vi "MacroExecution and Timing.vi"(7 "MacroExecution and Timing Command":T3, 8 "Error In":errorcluster, 10 "Index IN":i32, 11 "Macro IN":string[](array[string])) -> (0 "Error Out":errorcluster, 1 "Estimated Timing cluster":T1, 2 "Pause Duration":dbl, 3 "Execution Status":T2=enum."Skip", 4 "Current Command":string, 5 "Current Execution Index":i32)   [LabVIEW 2012]
doc: "SciScan 1.2 160622"
uses:
  Macro Execution and Timing_Commands.ctl
  Custom Controls and Typedefs/ExecutionStatus.ctl
  Estimated Timing Cluster.ctl
  Custom Controls/MAIN Image panel tab Control type def.ctl
  MacroGUI Module/Custom Controls and Typedefs/LOOP Control Cluster.ctl
  Custom Controls/Stage Position Data.ctl
  Custom Controls/file format type def.ctl
  GFG/GFGbooleanGet.vi
  GFG/GFGpathGet.vi
  GFG/GFG library.lvlib
panel:
  out "Step time array":dbl[](array[numeric])
  out "Remaining/Estimated Run Time":dbl
  out "Skip?":bool
  out "Paused?":bool
  out "Execution Complete?":bool
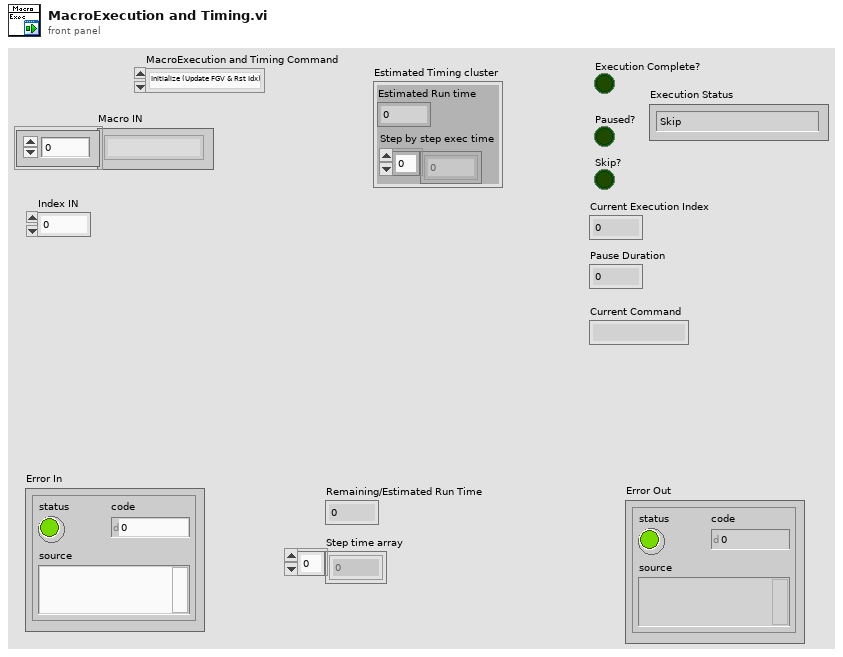
[diagram p1: front panel]
types:
  T1 = typedef "Estimated Timing Cluster.ctl" = cluster{"Estimated Run time":dbl, "Step by step exec time":dbl[]}
  T2 = typedef "ExecutionStatus.ctl" = enum16{"Instruction Available", "Skip", "Exec Paused", "Exec Complete", "Exec Waiting for Trigger"}
  T3 = typedef "Macro Execution and Timing_Commands.ctl" = enum16{"Initialize (Update FGV & Rst Idx)", "Run", "EstimateTime", "Preview", "Update Macro array (Idx Unchanged)", "Update Index", "Clear Timing Info"}
  T4 = typedef "MAIN Image panel tab Control type def.ctl" = enum32{"Channel 1", "Channel 2", "Channel 3", "Channel 4", "all channels", "RGB overlay", "ROI", "arbitrary line scan"}
  T5 = typedef "LOOP Control Cluster.ctl" = cluster{"Index of LOOP.Start":i32, "Iteration Count Down":i32, "No of iterations (N)":i32}
  T6 = typedef "file format type def.ctl" = enum16{"16bit raw", "32bit raw", "16bit multi-tiff (interleave)", "16bit multi-tiff (separate)", "16bit multi-tiff (stacked)", "32bit multi-tiff (interleave)", "32bit multi-tiff (separate)", "32bit multi-tiff (stacked)", "16bit tiff series (interleave)", "16bit tiff series (separate)", "16bit tiff series (stacked)", "32bit tiff series (interleave)", "32bit tiff series (separate)", "32bit tiff series (stacked)"}
  T7 = typedef "Stage Position Data.ctl" = cluster{"X":dbl, "Y":dbl, "Z":dbl}
  T8 = typedef "Macro_Action_List.ctl" = enum16{"Unknown Command", "2D.Frame.Scan", "2D.Line.Scan", "Load.Settings.File", "Move.To.Position", "Pause", "Z.Stack", "LOOP.Start", "LOOP.End", "Record", "Fast.Z", "Generic", "Slow.Z", "Tiling", "Preset.End"}
  T9 = typedef "VariantType.lvlib/Type.ctl" = enum8{"Invalid Type", "Void", "I8", "I16", "I32", "I64", "U8", "U16", "U32", "U64", "Single Float", "Double Float", "Extended Float", "Single Complex", "Double Complex", "Extended Complex", "Enum U8", "Enum U16", "Enum U32", "Enum U64", "Single Float With Unit", "Double Float With Unit", "Extended Float With Unit", "Single Complex with Unit", "Double Complex with Unit", "Extended Complex with Unit", "Boolean", "String", "Path", "Picture", "Tag", "Array", "Cluster", "Variant", "LV Variant", "Waveform", "Timestamp", "Digital Waveform", "Digital Data", "ExpressData", "Refnum", "External Data", "VI", "Poly VI", "LabVIEW Class Instance", "Fixed Point"}
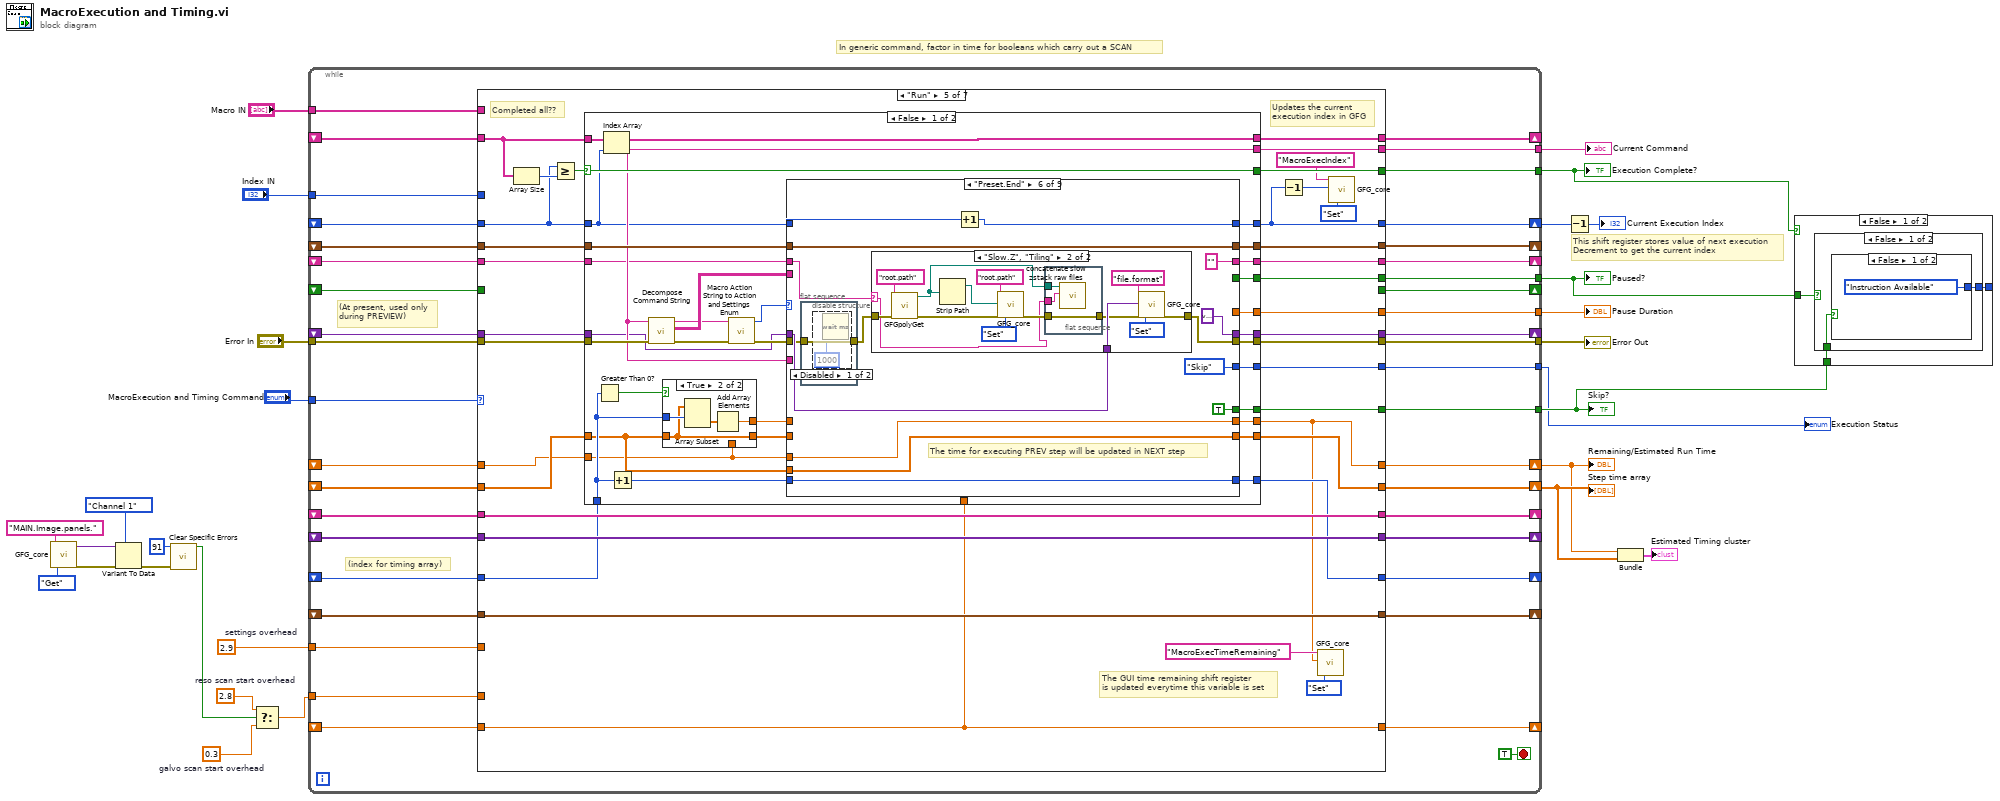
[diagram p0: block diagram]
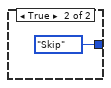
[diagram p2: hidden frame]
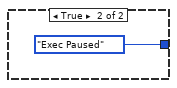
[diagram p3: hidden frame]
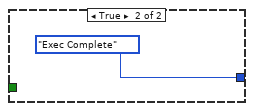
[diagram p4: hidden frame]
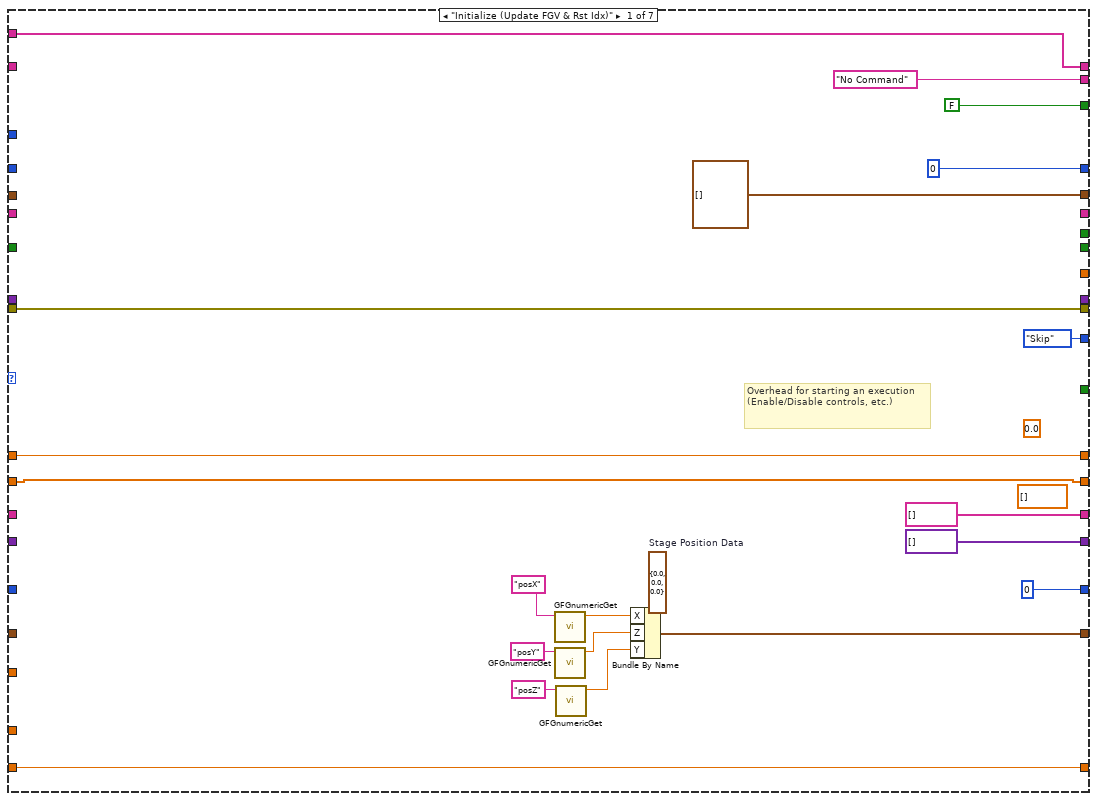
[diagram p5: hidden frame]
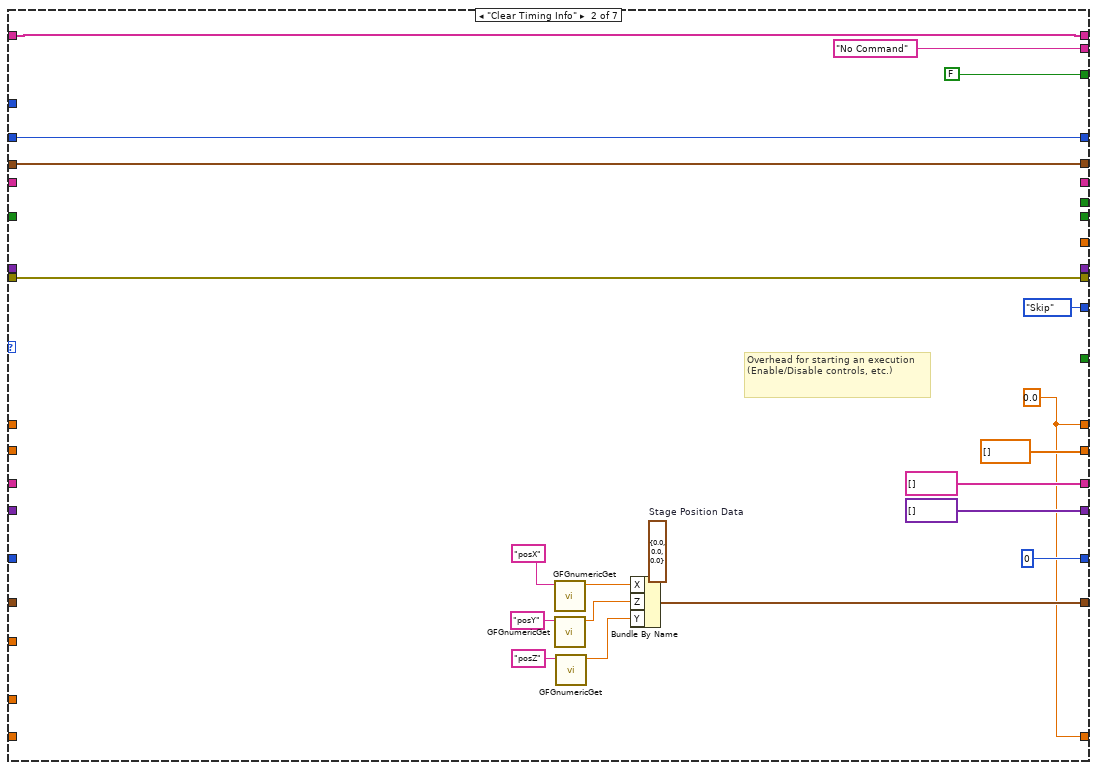
[diagram p6: hidden frame]
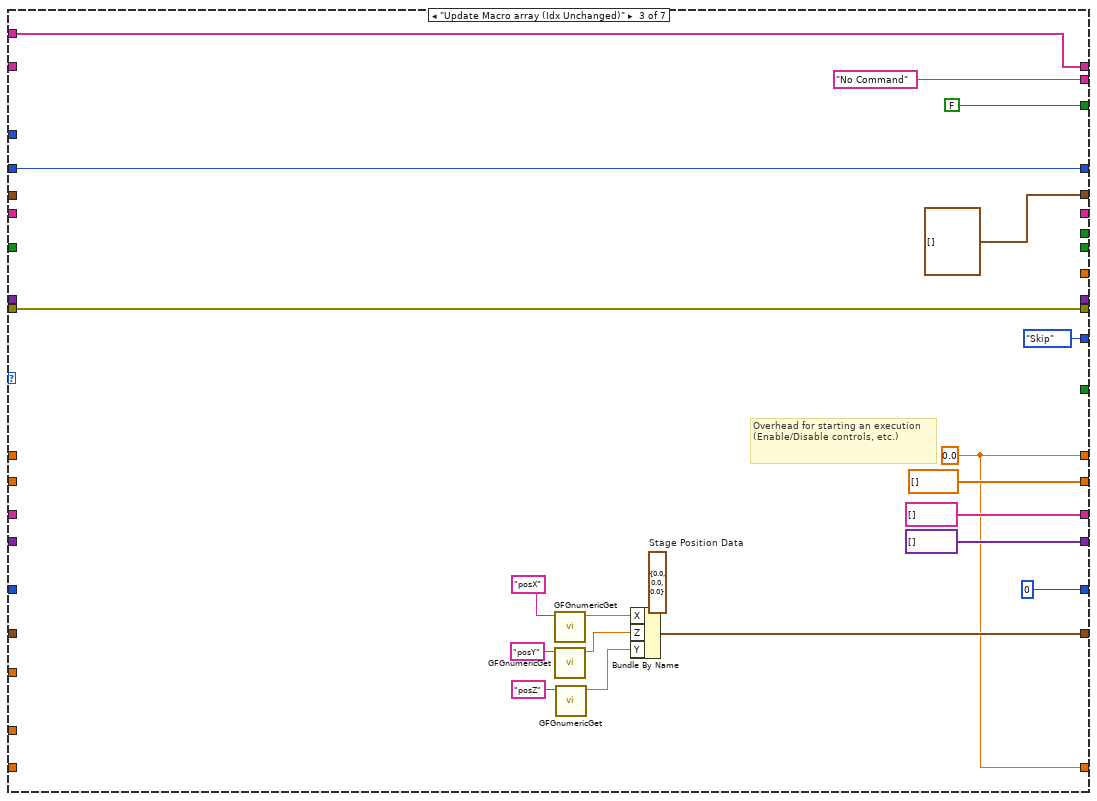
[diagram p7: hidden frame]
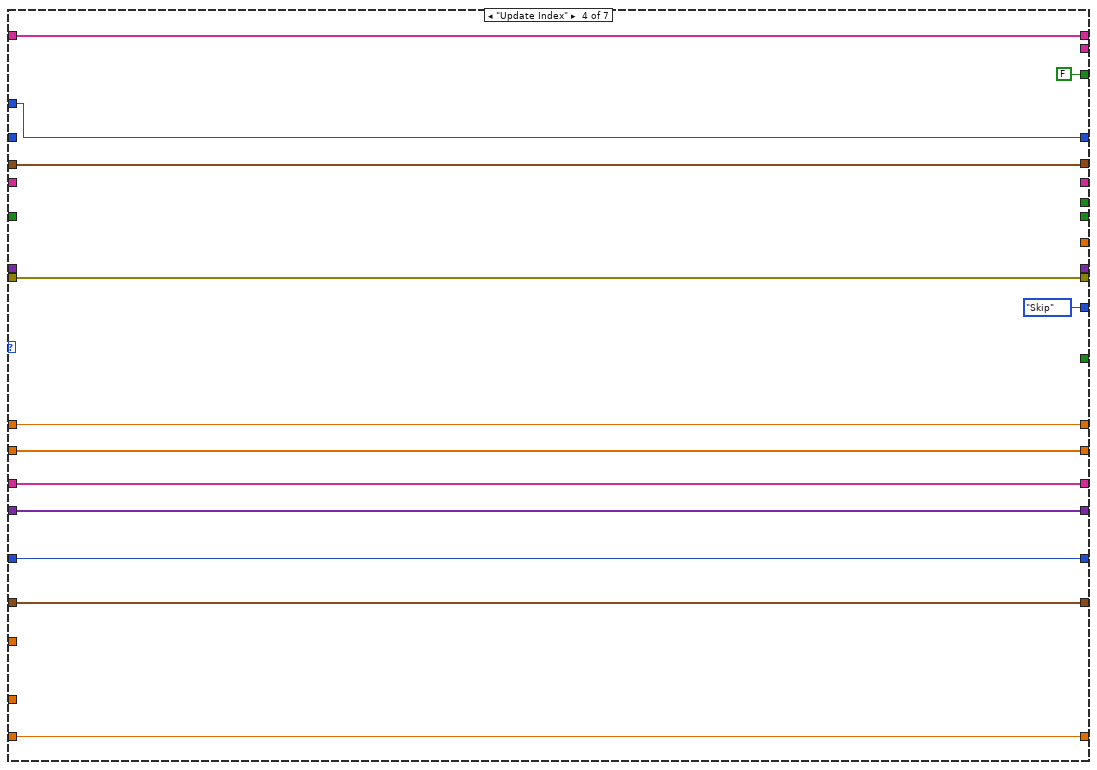
[diagram p8: hidden frame]
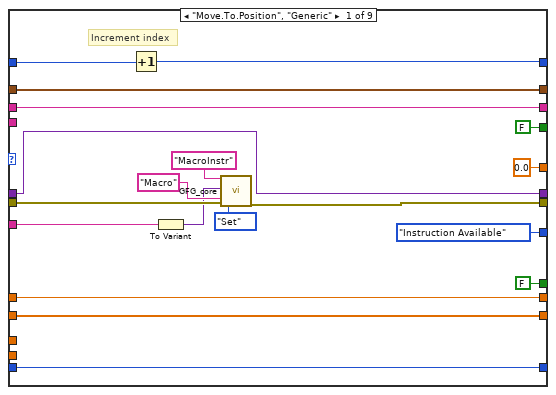
[diagram p10: hidden frame]
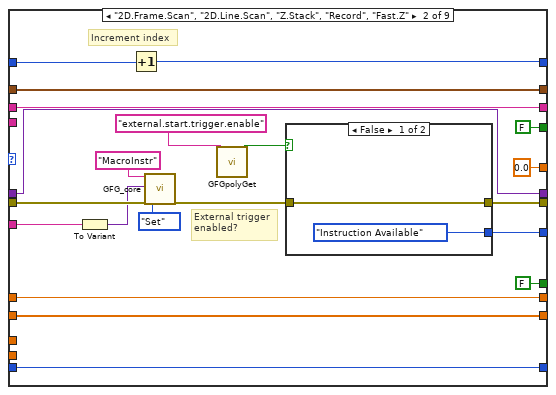
[diagram p11: hidden frame]
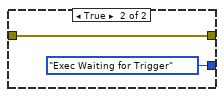
[diagram p12: hidden frame]
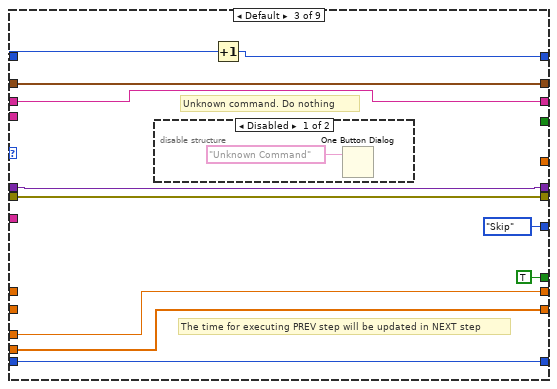
[diagram p13: hidden frame]
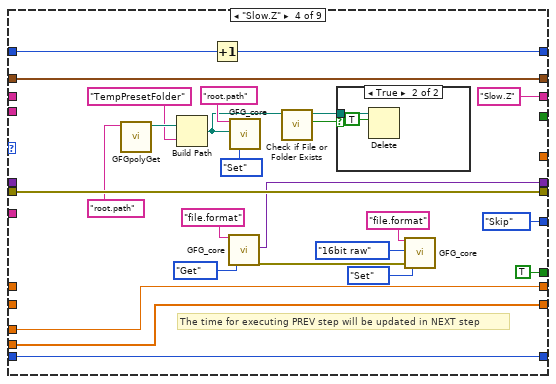
[diagram p15: hidden frame]
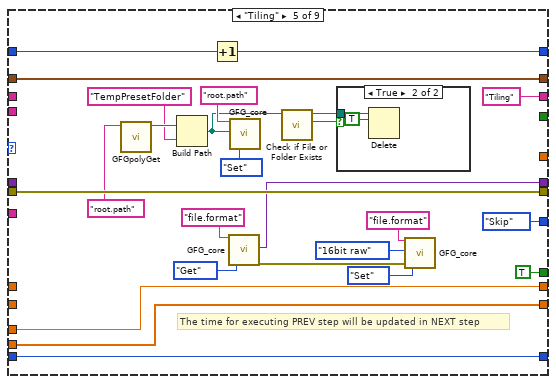
[diagram p17: hidden frame]
diagram:
  w9 = 0.3  # galvo scan start overhead
  w11 = 2.8  # reso scan start overhead
  w12 = 2.9  # settings overhead
  # "In generic command, factor in time for booleans which carry out a SCAN"
  # "This shift register stores value of next execution\nDecrement to get the current index"
  n1 = call "GFG_core.vi"("Variable Name in"="MAIN.Image.panels.", "Action"=enum16{"Init", "Set", "Get", "Clear"}."Get") -> ("Variant Out"=w5:variant, "error out"=w7:errorcluster)  [unwired: 11 in, 5 out]
  n2 = Variant To Data(error in=w7, type=MAIN_Image_panel_tab_Control_type_def."Channel 1" ("MAIN Image panels"), Variant=w5) -> (error out=w4:errorcluster)  [unwired: 1 out]
  n3 = call "Clear Specific Errors.vi"("Error In"=w4, "Error number In"=91) -> ("Error Cleared?"=w2:bool)  [unwired: 8 in, 1 out]
  n4 = Select(t=w11, s=w2, f=w9) -> (s? t:f=w10:dbl)
  n5 = while {
    shift-right: [w63] -> w24
    shift-left: _ -> [w68]
    tunnel: [w65] -> w22
    tunnel: "MacroExecution and Timing Command" -> [w64]
    shift-right: [w62] -> _
    shift-left: _ -> [w67]
    shift-right: [w60] -> _
    shift-left: _ -> [w61]
    tunnel: "Error In" -> [w59]
    tunnel: [w58] -> w26
    tunnel: [w57] -> w21
    tunnel: [w56] -> w25
    tunnel: [w55] -> w20
    tunnel: [w54] -> w23
    shift-right: [w53] -> w17
    shift-left: _ -> [w52]
    shift-right: [w51] -> w18
    shift-left: _ -> [w50]
    shift-right: [w49] -> _
    shift-left: _ -> [w47]
    shift-right: [w48] -> _
    shift-left: _ -> [w46]
    shift-right: [w45] -> _
    shift-left: _ -> [w44]
    shift-right: [w43] -> _
    shift-left: _ -> [w42]
    shift-right: [w41] -> _
    shift-left: _ -> [w40]
    tunnel: [w39] -> w15
    tunnel: "Macro IN" -> [w38]
    tunnel: "Index IN" -> [w37]
    tunnel: w12 -> [w36]
    tunnel: w10 -> [w35]
    shift-right: [w34] -> _
    shift-left: _ -> [w33]
    shift-right: [w32] -> _
    shift-left: _ -> [w31]
    shift-right: [w30] -> _
    shift-left: _ -> [w29]
    stop <- TRUE stop-if-true
    # "(At present, used only\nduring PREVIEW)"
    # "(index for timing array)"
    n6 = case shown="\"Run\"" w64 {
      tunnel: w68 -> [_ w92 w110 _ w176 w472 w907]
      tunnel: w67 -> [_ w94 _ w142 w175 w471 w920]
      tunnel: [FALSE FALSE FALSE FALSE w173 w469 w917] -> w65
      tunnel: [0 w92 w110 w139 w160 w464 w918] -> w63
      tunnel: [w72 w94 w111 w142 w172 w468 w920] -> w62
      tunnel: w61 -> [_ w93 _ w138 w171 w467 w911]
      tunnel: [T5[] [] w93 T5[] [] w138 w169 w465 w911] -> w60
      tunnel: w59 -> [w86 w108 w127 w137 w170 w466 w908]
      tunnel: [w86 w108 w127 w137 w168 w463 w910] -> w58
      tunnel: [_ _ _ _ w167 w462 _] -> w57
      tunnel: [_ _ _ _ w166 w461 _] -> w56
      tunnel: [_ _ _ _ w165 w460 _] -> w55
      tunnel: ["No Command" ("String") "No Command" ("String") "No Command" ("String") _ w164 w459 w916] -> w54
      tunnel: [w70 w90 w113 w141 w149 w458 w924] -> w53
      tunnel: w52 -> [w70 _ _ w141 w147 w457 w924]
      tunnel: [w71 dbl[] [] dbl[] [] w135 w154 w456 w923] -> w51
      tunnel: w50 -> [w71 _ _ w135 w156 w455 w923]
      tunnel: [string[] [] string[] [] string[] [] w134 w163 w452 w915] -> w49
      tunnel: [variant[] [] variant[] [] variant[] [] w133 w162 w451 w914] -> w48
      tunnel: w47 -> [_ _ _ w134 w163 w454 w915]
      tunnel: w46 -> [_ _ _ w133 w162 w453 w914]
      tunnel: [w75 w97 w115 w131 w161 w449 w912] -> w45
      tunnel: w44 -> [_ _ _ w131 w161 w450 w912]
      tunnel: [0 0 0 w132 w153 0 w913] -> w43
      tunnel: w42 -> [_ _ _ w132 w155 _ w913]
      tunnel: [w69 w90 w113 w130 w152 w448 w909] -> w41
      tunnel: w40 -> [w69 _ _ w130 w152 w447 w909]
      tunnel: [ExecutionStatus."Skip" ("Execution Status") ExecutionStatus."Skip" ("Execution Status") ExecutionStatus."Skip" ("Execution Status") ExecutionStatus."Skip" ("Execution Status") w148 w445 w919] -> w39
      tunnel: w38 -> [w72 _ w111 _ _ _ _]
      tunnel: w37 -> [_ _ _ w139 _ _ _]
      tunnel: w36 -> [_ _ _ _ _ w444 _]
      tunnel: w35 -> [_ _ _ _ _ w443 _]
      tunnel: [_ _ _ _ w146 _ _] -> w34
      tunnel: w33 -> [_ _ _ _ w145 _ _]
      tunnel: [_ _ _ _ w144 _ _] -> w32
      tunnel: w31 -> [_ _ _ _ w143 _ _]
      tunnel: [_ _ _ _ _ _ w906] -> w30
      tunnel: w29 -> [_ _ _ _ _ _ w905]
      frame "Initialize (Update FGV & Rst Idx)" {
        w79 = T7 {"X"=0.0, "Y"=0.0, "Z"=0.0}  # Stage Position Data
        (unwired) dbl[] []
        (unwired) 0.0 ("number")
        # "Overhead for starting an execution\n(Enable/Disable controls, etc.)"
        n7 = call "GFGnumericGet.vi"("Variable Name in"="posX" ("String")) -> ("Numeric"=w78:dbl)  [unwired: 8 in, 2 out]
        n8 = call "GFGnumericGet.vi"("Variable Name in"="posY" ("String")) -> ("Numeric"=w77:dbl)  [unwired: 8 in, 2 out]
        n9 = call "GFGnumericGet.vi"("Variable Name in"="posZ" ("String")) -> ("Numeric"=w76:dbl)  [unwired: 8 in, 2 out]
        n10 = Bundle By Name(cluster=w79, "X"=w78, "Z"=w77, "Y"=w76) -> (w75:T7)
      }
      frame "Clear Timing Info" {
        w101 = T7 {"X"=0.0, "Y"=0.0, "Z"=0.0}  # Stage Position Data
        w90 = 0.0 ("number")
        # "Overhead for starting an execution\n(Enable/Disable controls, etc.)"
        n11 = call "GFGnumericGet.vi"("Variable Name in"="posX" ("String")) -> ("Numeric"=w100:dbl)  [unwired: 8 in, 2 out]
        n12 = call "GFGnumericGet.vi"("Variable Name in"="posY" ("String")) -> ("Numeric"=w99:dbl)  [unwired: 8 in, 2 out]
        n13 = call "GFGnumericGet.vi"("Variable Name in"="posZ" ("String")) -> ("Numeric"=w98:dbl)  [unwired: 8 in, 2 out]
        n14 = Bundle By Name(cluster=w101, "X"=w100, "Z"=w99, "Y"=w98) -> (w97:T7)
      }
      frame "Update Macro array (Idx Unchanged)" {
        w119 = T7 {"X"=0.0, "Y"=0.0, "Z"=0.0}  # Stage Position Data
        w113 = 0.0 ("number")
        # "Overhead for starting an execution\n(Enable/Disable controls, etc.)"
        n15 = call "GFGnumericGet.vi"("Variable Name in"="posX" ("String")) -> ("Numeric"=w118:dbl)  [unwired: 8 in, 2 out]
        n16 = call "GFGnumericGet.vi"("Variable Name in"="posY" ("String")) -> ("Numeric"=w117:dbl)  [unwired: 8 in, 2 out]
        n17 = call "GFGnumericGet.vi"("Variable Name in"="posZ" ("String")) -> ("Numeric"=w116:dbl)  [unwired: 8 in, 2 out]
        n18 = Bundle By Name(cluster=w119, "X"=w118, "Z"=w117, "Y"=w116) -> (w115:T7)
      }
      frame "Update Index" {
      }
      frame "Run" {
        # "Updates the current\nexecution index in GFG"
        # "The GUI time remaining shift register\nis updated everytime this variable is set"
        # "Completed all??"
        n19 = Array Size(array=w175) -> (size(s)=w177:i32)
        n20 = Greater Or Equal?(x=w176, y=w177) -> (x >= y?=w174:bool)
        n21 = case shown="False" w174 {
          selector: w174 -> [w209 w441]
          tunnel: w176 -> [w197 w438]
          tunnel: w175 -> [w208 w442]
          tunnel: [w209 w441] -> w173
          tunnel: [w208 w442] -> w172
          tunnel: w171 -> [w206 w439]
          tunnel: w170 -> [w207 w440]
          tunnel: [w205 w439] -> w169
          tunnel: [w204 w438] -> w160
          tunnel: [w203 w440] -> w168
          tunnel: [w201 _] -> w167
          tunnel: [w200 _] -> w166
          tunnel: [w199 _] -> w165
          tunnel: [w198 "No Command" ("String")] -> w164
          tunnel: w156 -> [w187 w435]
          tunnel: w155 -> [w190 _]
          tunnel: [w196 w435] -> w154
          tunnel: [w195 w434] -> w149
          tunnel: [w194 0] -> w153
          tunnel: w152 -> [_ w434]
          tunnel: [w193 ExecutionStatus."Exec Complete" ("Execution Status")] -> w148
          tunnel: w147 -> [w186 _]
          tunnel: [w181 _] -> w146
          tunnel: w145 -> [w180 _]
          tunnel: [w179 _] -> w144
          tunnel: w143 -> [w178 _]
          frame False {
            n22 = Greater Than 0?(x=w190) -> (x > 0?=w191:bool)
            n23 = Index Array(array=w208, index=w197) -> (element=w198:string)
            n24 = Increment(x=w190) -> (x+1=w192:i32)
            n25 = call "Decompose Command String.vi"("Error In"=w207, "Command IN"=w198) -> ("Error Out"=w185:errorcluster, "Parameter Table"=w202:string[][], "Action"=w183:string)  [unwired: 6 in, 1 out]
            n26 = case shown="True" w191 {
              tunnel: w187 -> [w211 w213]
              tunnel: w190 -> [_ w215]
              tunnel: [w211 w213] -> w189
              tunnel: [w210 w212] -> w188
              tunnel: w186 -> [w210 _]
              frame False {
              }
              frame True {
                n27 = Array Subset(array=w213, index=w215) -> (w214:dbl[])  [unwired: 1 in]
                n28 = Add Array Elements(numeric array=w214) -> (sum=w212:dbl)
              }
            }
            n29 = call "Macro Action String to Action and Settings Enum.vi"("error in (no error)"=w185, "Action String IN"=w183) -> ("error out"=w184:errorcluster, "Action Enum OUT"=w182:T8)  [unwired: 6 in, 2 out]
            n30 = case shown="\"Preset.End\"" w182 {
              tunnel: w184 -> [w225 w247 w267 w293 w320 w327 w368 w390 w415]
              tunnel: w197 -> [w234 w255 w270 w296 w323 w340 w376 w392 w412]
              tunnel: w206 -> [w232 w253 w268 w294 w321 w338 w377 w395 w417]
              tunnel: [w232 w253 w268 w294 w321 w338 w377 w394 w416] -> w205
              tunnel: [w233 w254 w269 w295 w322 w339 w375 w391 w411] -> w204
              tunnel: [w222 w240 w267 w293 w320 w328 w368 w390 w415] -> w203
              tunnel: w198 -> [w224 w246 _ _ _ _ _ _ _]
              tunnel: w202 -> [_ _ _ _ _ _ w373 w389 _]
              tunnel: [FALSE FALSE _ _ _ _ TRUE _ _] -> w201
              tunnel: [0.0 0.0 _ _ _ _ w369 _ _] -> w200
              tunnel: [FALSE ("Skip?") FALSE ("Skip?") TRUE ("Skip?") TRUE ("Skip?") TRUE ("Skip?") TRUE ("Skip?") FALSE ("Skip?") TRUE ("Skip?") TRUE ("Skip?")] -> w199
              tunnel: w188 -> [w219 w238 _ _ _ _ w364 w381 w403]
              tunnel: w189 -> [w220 w239 _ _ _ _ w365 w382 w404]
              tunnel: [w220 w239 w263 w289 w316 w334 w365 w382 w404] -> w196
              tunnel: [w219 w238 w262 w288 w315 w333 w364 w381 w403] -> w195
              tunnel: [w218 w237 w264 w290 w317 w335 w363 w380 w402] -> w194
              tunnel: [ExecutionStatus."Instruction Available" ("Execution Status") w241 ExecutionStatus."Skip" ("Execution Status") ExecutionStatus."Skip" ("Execution Status") ExecutionStatus."Skip" ("Execution Status") ExecutionStatus."Skip" ("Execution Status") ExecutionStatus."Exec Paused" ("Execution Status") ExecutionStatus."Skip" ("Execution Status") ExecutionStatus."Skip" ("Execution Status")] -> w193
              tunnel: w192 -> [w218 w237 w264 w290 w317 w335 w363 w380 w402]
              tunnel: w187 -> [_ _ w263 w289 w316 w334 _ _ _]
              tunnel: w186 -> [_ _ w262 w288 w315 w333 _ _ _]
              tunnel: [w217 w236 w261 "Slow.Z" ("Variable Name in") "Tiling" ("Variable Name in") "" ("Variable Name in") w362 w379 w401] -> w181
              tunnel: w180 -> [w217 w236 w261 _ _ w331 w362 w379 w401]
              tunnel: [w216 w235 w260 w276 w303 variant ("Variant Out") w361 w378 w400] -> w179
              tunnel: w178 -> [w216 w235 w260 _ _ w329 w361 w378 w400]
              frame "Move.To.Position", "Generic" {
                # "Increment index"
                n31 = Increment(x=w234) -> (x+1=w233:i32)
                n32 = To Variant(anything=w224) -> (Variant=w223:variant)
                n33 = call "GFG_core.vi"("Variable Name in"="MacroInstr" ("Source VI"), "Variant in"=w223, "Source VI"="Macro", "error in (no error)"=w225, "Action"=enum16{"Init", "Set", "Get", "Clear"}."Set") -> ("error out"=w222:errorcluster)  [unwired: 8 in, 6 out]
              }
              frame "2D.Frame.Scan", "2D.Line.Scan", "Z.Stack", "Record", "Fast.Z" {
                # "External trigger \nenabled?"
                # "Increment index"
                n34 = To Variant(anything=w246) -> (Variant=w245:variant)
                n35 = Increment(x=w255) -> (x+1=w254:i32)
                n36 = call "GFG_core.vi"("Variable Name in"="MacroInstr" ("Source VI"), "Variant in"=w245, "error in (no error)"=w247, "Action"=enum16{"Init", "Set", "Get", "Clear"}."Set") -> ("error out"=w242:errorcluster)  [unwired: 9 in, 6 out]
                n37 = call-poly "GFGpolyGet.vi"("Variable Name in"="external.start.trigger.enable") -> ("Boolean Value OUT"=w243:bool)  [unwired: 9 in, 1 out]
                n38 = case shown="False" w243 {
                  tunnel: w242 -> [w256 w258]
                  tunnel: [ExecutionStatus."Instruction Available" ("Execution Status") ExecutionStatus."Exec Waiting for Trigger" ("Execution Status")] -> w241
                  tunnel: [w256 w258] -> w240
                  frame False {
                  }
                  frame True {
                  }
                }
              }
              frame Default {
                # "The time for executing PREV step will be updated in NEXT step"
                # "Unknown command. Do nothing"
                n39 = disable-structure shown="Disabled" {
                  frame Disabled {
                    n40 = One Button Dialog(message="Unknown Command") -> ()  [unwired: 1 in, 1 out]
                  }
                  frame Enabled {
                  }
                }
                n41 = Increment(x=w270) -> (x+1=w269:i32)
              }
              frame "Slow.Z" {
                # "The time for executing PREV step will be updated in NEXT step"
                n42 = call-poly "GFGpolyGet.vi"("Variable Name in"="root.path") -> ("Path"=w283:path)  [unwired: 8 in, 2 out]
                n43 = Build Path(base path=w283, name or relative path="TempPresetFolder") -> (appended path=w274:path)
                n44 = Increment(x=w296) -> (x+1=w295:i32)
                n45 = call "GFG_core.vi"("Variable Name in"="file.format", "Action"=enum16{"Init", "Set", "Get", "Clear"}."Get") -> ("Variant Out"=w276:variant, "error out"=w275:errorcluster)  [unwired: 11 in, 5 out]
                n46 = call "GFG_core.vi"("Variable Name in"="root.path", "Variant in"=w274, "Action"=enum16{"Init", "Set", "Get", "Clear"}."Set") -> ()  [unwired: 10 in, 7 out]
                n47 = call <vilib>:"Check if File or Folder Exists.vi"("path"=w274) -> ("file or folder exists?"=w273:bool, "dup path"=w272:path)  [unwired: 8 in, 1 out]
                n48 = case shown="True" w273 {
                  tunnel: w272 -> [_ w298]
                  frame False {
                  }
                  frame True {
                    n49 = Delete(path (use dialog)=w298, entire hierarchy (F)=TRUE) -> ()  [unwired: 3 in, 3 out]
                  }
                }
                n50 = call "GFG_core.vi"("Variable Name in"="file.format", "Variant in"=file_format_type_def."16bit raw" ("file format"), "error in (no error)"=w275, "Action"=enum16{"Init", "Set", "Get", "Clear"}."Set") -> ()  [unwired: 9 in, 7 out]
              }
              frame "Tiling" {
                # "The time for executing PREV step will be updated in NEXT step"
                n51 = call-poly "GFGpolyGet.vi"("Variable Name in"="root.path") -> ("Path"=w310:path)  [unwired: 8 in, 2 out]
                n52 = Build Path(base path=w310, name or relative path="TempPresetFolder") -> (appended path=w301:path)
                n53 = Increment(x=w323) -> (x+1=w322:i32)
                n54 = call "GFG_core.vi"("Variable Name in"="file.format", "Action"=enum16{"Init", "Set", "Get", "Clear"}."Get") -> ("Variant Out"=w303:variant, "error out"=w302:errorcluster)  [unwired: 11 in, 5 out]
                n55 = call "GFG_core.vi"("Variable Name in"="root.path", "Variant in"=w301, "Action"=enum16{"Init", "Set", "Get", "Clear"}."Set") -> ()  [unwired: 10 in, 7 out]
                n56 = call <vilib>:"Check if File or Folder Exists.vi"("path"=w301) -> ("file or folder exists?"=w300:bool, "dup path"=w299:path)  [unwired: 8 in, 1 out]
                n57 = case shown="True" w300 {
                  tunnel: w299 -> [_ w325]
                  frame False {
                  }
                  frame True {
                    n58 = Delete(path (use dialog)=w325, entire hierarchy (F)=TRUE) -> ()  [unwired: 3 in, 3 out]
                  }
                }
                n59 = call "GFG_core.vi"("Variable Name in"="file.format", "Variant in"=file_format_type_def."16bit raw" ("file format"), "error in (no error)"=w302, "Action"=enum16{"Init", "Set", "Get", "Clear"}."Set") -> ()  [unwired: 9 in, 7 out]
              }
              frame "Preset.End" {
                # "The time for executing PREV step will be updated in NEXT step"
                n60 = flat-sequence {
                  tunnel: w327 -> [w341]
                  tunnel: [w341] -> w326
                  frame #0 {
                    n61 = disable-structure shown="Disabled" {
                      frame Disabled {
                        n62 = Wait (ms)(milliseconds to wait=u32 1000) -> ()  [unwired: 1 out]
                      }
                      frame Enabled {
                      }
                    }
                  }
                }
                n63 = case shown="\"Slow.Z\", \"Tiling\"" w331 {
                  selector: w331 -> [_ w344]
                  tunnel: w329 -> [_ w348]
                  tunnel: [w343 w346] -> w328
                  tunnel: w326 -> [w343 w345]
                  frame Default {
                  }
                  frame "Slow.Z", "Tiling" {
                    n64 = call-poly "GFGpolyGet.vi"("error in (no error)"=w345, "Variable Name in"="root.path") -> ("error out"=w357:errorcluster, "Path"=w351:path)  [unwired: 7 in, 1 out]
                    n65 = Strip Path(path=w351) -> (stripped path=w356:path)  [unwired: 1 out]
                    n66 = call "GFG_core.vi"("Variable Name in"="root.path", "Variant in"=w356, "error in (no error)"=w357, "Action"=enum16{"Init", "Set", "Get", "Clear"}."Set") -> ("error out"=w352:errorcluster)  [unwired: 9 in, 6 out]
                    n67 = flat-sequence {
                      tunnel: w352 -> [w359]
                      tunnel: w351 -> [w360]
                      tunnel: [w359] -> w347
                      tunnel: w344 -> [w358]
                      frame #0 {
                        n68 = call "concatenate slow zstack raw files.vi"("preset type"=w358, "slow z root folder"=w360) -> ()  [unwired: 10 in]
                      }
                    }
                    n69 = call "GFG_core.vi"("Variable Name in"="file.format", "Variant in"=w348, "error in (no error)"=w347, "Action"=enum16{"Init", "Set", "Get", "Clear"}."Set") -> ("error out"=w346:errorcluster)  [unwired: 9 in, 6 out]
                  }
                }
                n70 = Increment(x=w340) -> (x+1=w339:i32)
              }
              frame "Pause" {
                # "Update Remaining time\nwhen PREV step completes"
                n71 = Increment(x=w376) -> (x+1=w375:i32)
                n72 = Index Array(array=w373, index (row)=0, index (col)=1 ("disabled index (col)")) -> (element=w370:string)
                n73 = Fract/Exp String To Number(string=w370) -> (number=w369:dbl)  [unwired: 3 in, 1 out]
              }
              frame "LOOP.Start" {
                # "Increment index"
                # "Insert loop details into index 0"
                # "Get no. of iterations from the arguments of LOOP.Start"
                n74 = Index Array(array=w389, index (row)=0, index (col)=1 ("disabled index (col)")) -> (element=w396:string)
                n75 = Decimal String To Number(string=w396) -> (number=w387:i32)  [unwired: 2 in, 1 out]
                n76 = Bundle By Name(cluster=T5 {"Index of LOOP.Start"=0, "Iteration Count Down"=0, "No of iterations (N)"=0} ("LOOP Control Cluster"), "Index of LOOP.Start"=w392, "Iteration Count Down"=w387, "No of iterations (N)"=w387) -> (w384:T5)
                n77 = Increment(x=w392) -> (x+1=w391:i32)
                n78 = Insert Into Array(array=w395, index=0, new element=w384) -> (w394:T5[])
                n79 = call "GFG_core.vi"("Variable Name in"="MacroLoopUpdate", "Variant in"=w384, "Action"=enum16{"Init", "Set", "Get", "Clear"}."Set") -> ()  [unwired: 10 in, 7 out]
              }
              frame "LOOP.End" {
                # "Set GFG Variable to update GUI"
                # "Determine next index"
                # "completed iterations?"
                n80 = Index Array(array=w417, index=0) -> (element=w414:T5)
                n81 = Unbundle By Name(w414) -> ("Index of LOOP.Start"=w410:i32, "Iteration Count Down"=w419:i32)
                n82 = Decrement(x=w419) -> (x-1=w413:i32)
                n83 = Less Or Equal To 0?(x=w413) -> (x <= 0?=w418:bool)
                n84 = Bundle(cluster=w414, "Index of LOOP.Start"=w410, "Iteration Count Down"=w413) -> (w407:T5)  [unwired: 1 in]
                n85 = case shown="True" w418 {
                  tunnel: w417 -> [w426 w432]
                  tunnel: [w423 w431] -> w416
                  tunnel: w407 -> [w424 _]
                  tunnel: w412 -> [_ w428]
                  tunnel: [w421 w427] -> w411
                  tunnel: w410 -> [w422 _]
                  frame False {
                    n86 = Increment(x=w422) -> (x+1=w421:i32)
                    n87 = Replace Array Subset(array=w426, new element=w424, index=0) -> (w423:T5[])
                  }
                  frame True {
                    n88 = Increment(x=w428) -> (x+1=w427:i32)
                    n89 = Delete From Array(array=w432, length=1, index=0) -> (array with subset deleted=w431:T5[])  [unwired: 1 out]
                  }
                }
                n90 = call "GFG_core.vi"("Variable Name in"="MacroLoopUpdate", "Variant in"=w407, "Action"=enum16{"Init", "Set", "Get", "Clear"}."Set") -> ()  [unwired: 10 in, 7 out]
              }
            }
          }
          frame True {
            # "Nothing more to executed.\nRemaining time =  Estimated Time"
            # "Reset commnds executed to 0"
            # "Finished Running"
          }
        }
        n91 = Decrement(x=w160) -> (x-1=w157:i32)
        n92 = call "GFG_core.vi"("Variable Name in"="MacroExecTimeRemaining", "Variant in"=w149, "Action"=enum16{"Init", "Set", "Get", "Clear"}."Set") -> ()  [unwired: 10 in, 7 out]
        n93 = call "GFG_core.vi"("Variable Name in"="MacroExecIndex", "Variant in"=w157, "Action"=enum16{"Init", "Set", "Get", "Clear"}."Set") -> ()  [unwired: 10 in, 7 out]
      }
      frame "EstimateTime" {
        # "Completed all??"
        n94 = Array Size(array=w471) -> (size(s)=w473:i32)
        n95 = Greater Or Equal?(x=w472, y=w473) -> (x >= y?=w470:bool)
        n96 = case shown="False" w470 {
          selector: w470 -> [w504 w900]
          tunnel: w472 -> [w474 _]
          tunnel: w471 -> [w475 w901]
          tunnel: [w504 w900] -> w469
          tunnel: [w475 w901] -> w468
          tunnel: w467 -> [w502 w898]
          tunnel: w466 -> [w503 w899]
          tunnel: [w501 w898] -> w465
          tunnel: [w500 0] -> w464
          tunnel: [w499 w899] -> w463
          tunnel: [w497 _] -> w462
          tunnel: [w496 _] -> w461
          tunnel: [w495 _] -> w460
          tunnel: [w478 "No Command" ("String")] -> w459
          tunnel: [w494 w890] -> w458
          tunnel: w457 -> [w493 w890]
          tunnel: [w492 w891] -> w456
          tunnel: w455 -> [w491 w891]
          tunnel: w454 -> [w490 w894]
          tunnel: w453 -> [w489 w893]
          tunnel: [w488 w894] -> w452
          tunnel: [w487 w893] -> w451
          tunnel: w450 -> [w486 w896]
          tunnel: [w485 w896] -> w449
          tunnel: [w484 w890] -> w448
          tunnel: w447 -> [w484 _]
          tunnel: [ExecutionStatus."Skip" ("Execution Status") ExecutionStatus."Exec Complete" ("Execution Status")] -> w445
          tunnel: w444 -> [w477 _]
          tunnel: w443 -> [w476 _]
          frame False {
            n97 = Index Array(array=w475, index=w474) -> (element=w478:string)
            n98 = call "Decompose Command String.vi"("Error In"=w503, "Command IN"=w478) -> ("Error Out"=w482:errorcluster, "Parameter Table"=w498:string[][], "Action"=w479:string)  [unwired: 6 in, 1 out]
            n99 = call "Macro Action String to Action and Settings Enum.vi"("error in (no error)"=w482, "Action String IN"=w479) -> ("error out"=w481:errorcluster, "Action Enum OUT"=w480:T8)  [unwired: 6 in, 2 out]
            n100 = case shown="\"Record\"" w480 {
              tunnel: w481 -> [w536 w553 w624 w643 w667 w708 w734 w760 w786 w808 w833 w863 w876 w889]
              tunnel: w474 -> [w542 w558 w627 w650 w670 w711 w737 w763 w789 w810 w830 w853 w866 w879]
              tunnel: w502 -> [w540 w557 w631 w651 w671 w712 w738 w764 w790 w813 w835 w851 w864 w877]
              tunnel: [w540 w557 w631 w651 w671 w712 w738 w764 w790 w812 w834 w851 w864 w877] -> w501
              tunnel: [w541 w543 w626 w649 w669 w710 w736 w762 w788 w809 w829 w852 w865 w878] -> w500
              tunnel: [w536 w553 w624 w643 w667 w708 w734 w760 w786 w808 w833 w863 w876 w889] -> w499
              tunnel: w498 -> [w534 w556 _ w647 _ _ _ _ _ w807 _ _ _ _]
              tunnel: [FALSE _ _ TRUE TRUE TRUE TRUE TRUE TRUE _ _ _ _ _] -> w497
              tunnel: [0.0 _ _ w641 _ _ _ _ _ _ _ _ _ _] -> w496
              tunnel: [FALSE ("Skip?") _ TRUE ("Skip?") FALSE ("Skip?") FALSE ("Skip?") FALSE ("Skip?") FALSE ("Skip?") FALSE ("Skip?") FALSE ("Skip?") TRUE ("Skip?") TRUE ("Skip?") TRUE ("Skip?") TRUE ("Skip?") TRUE ("Skip?")] -> w495
              tunnel: [w507 w548 w619 w638 w664 w705 w731 w757 w783 w797 w819 w855 w868 w881] -> w494
              tunnel: w493 -> [w508 w552 w623 w639 w665 w706 w732 w758 w784 w798 w820 w856 w869 w882]
              tunnel: [w518 w549 w620 w636 w663 w704 w730 w756 w782 w802 w824 w860 w873 w886] -> w492
              tunnel: w491 -> [w519 w551 w621 w635 w662 w703 w729 w755 w781 w803 w825 w861 w874 w887]
              tunnel: w490 -> [w517 w555 w630 w634 w661 w702 w728 w754 w780 w801 w823 w859 w872 w885]
              tunnel: w489 -> [w516 w554 w629 w633 w660 w701 w727 w753 w779 w800 w822 w858 w871 w884]
              tunnel: [w517 w547 w630 w634 w661 w702 w728 w754 w780 w801 w823 w859 w872 w885] -> w488
              tunnel: [w516 w546 w629 w633 w660 w701 w727 w753 w779 w800 w822 w858 w871 w884] -> w487
              tunnel: w486 -> [w512 w545 w628 w632 w659 w700 w726 w752 w778 w799 w821 w857 w870 w883]
              tunnel: [w512 w544 w628 w632 w659 w700 w726 w752 w778 w799 w821 w857 w870 w883] -> w485
              tunnel: w478 -> [_ _ _ _ _ w696 w722 w749 w774 _ _ _ _ _]
              tunnel: w477 -> [_ _ _ _ _ w694 w720 w746 w772 _ _ _ _ _]
              tunnel: w476 -> [_ _ _ _ w654 w692 w718 w744 w770 _ _ _ _ _]
              tunnel: w475 -> [_ _ _ _ w653 _ _ _ _ _ _ _ _ _]
              tunnel: w474 -> [_ _ _ _ w652 _ _ _ _ _ _ _ _ _]
              frame "Move.To.Position" {
                w532 = 1 ("index (row)")
                # "Total distance travelled"
                # "Time = Dist/Vel"
                # "Increment index"
                n101 = call "GFGnumericGet.vi"("Variable Name in"="stage.speed.slow" ("String")) -> ("Numeric"=w520:dbl)  [unwired: 8 in, 2 out]
                n102 = Index Array(array=w534, index (row) #1=0 ("index (row)"), index (col) #1=w532, index (row) #2=w532, index (col) #2=w532, index (row) #3=2 ("index (row)"), index (col) #3=w532) -> (element #1=w530:string, element #2=w529:string, element #3=w528:string)
                n103 = Increment(x=w542) -> (x+1=w541:i32)
                n104 = Fract/Exp String To Number(string=w530) -> (number=w527:dbl)  [unwired: 3 in, 1 out]
                n105 = Fract/Exp String To Number(string=w529) -> (number=w526:dbl)  [unwired: 3 in, 1 out]
                n106 = Fract/Exp String To Number(string=w528) -> (number=w525:dbl)  [unwired: 3 in, 1 out]
                n107 = Unbundle By Name(w512) -> ("X"=w515:dbl, "Z"=w514:dbl, "Y"=w513:dbl)
                n108 = Subtract(x=w526, y=w514) -> (x-y=w523:dbl)
                n109 = Subtract(x=w515, y=w527) -> (x-y=w524:dbl)
                n110 = Subtract(x=w525, y=w513) -> (x-y=w522:dbl)
                n111 = formula code="dist = sqrt(x*x+y*y+z*z);"("x"=w524, "y"=w523, "z"=w522) -> ("dist"=w521:dbl)
                n112 = Multiply(x=0.1, y=w520) -> (x*y=w506:dbl)
                n113 = Divide(x=w521, y=w506) -> (x/y=w510:dbl)
                n114 = Add(x=0.1, y=w510) -> (x+y=w509:dbl)
                n115 = Insert Into Array(array=w519, new element=w509) -> (w518:dbl[])  [unwired: 1 in]
                n116 = Add(x=w508, y=w509) -> (x+y=w507:dbl)
              }
              frame "Generic" {
                w550 = 0.1 ("y")
                # "overhead for generic command"
                n117 = for {
                  tunnel: w556 -> [w577] mode=indexing
                  shift-right: [w574] -> w547
                  shift-left: w555 -> [w576]
                  shift-right: [w573] -> w546
                  shift-left: w554 -> [w575]
                  shift-right: [w559] -> w544
                  shift-left: w545 -> [w569]
                  # "Stage positions\naffect the time\nfor move comnd.\n-- Store them!"
                  # "Is this a numeric\ndata type?"
                  n118 = Index Array(array=w577) -> (element #1=w565:string, element #2=w564:string)  [unwired: 2 in]
                  n119 = Equal?(x=w565, y="setX" ("element")) -> (x = y?=w563:bool)
                  n120 = Equal?(x=w565, y="setY" ("element")) -> (x = y?=w561:bool)
                  n121 = Equal?(x=w565, y="setZ" ("element")) -> (x = y?=w560:bool)
                  n122 = Fract/Exp String To Number(string=w564) -> (number=w562:dbl)  [unwired: 3 in, 1 out]
                  n123 = call "GFG_core.vi"("Variable Name in"=w565, "Action"=enum16{"Init", "Set", "Get", "Clear"}."Get") -> ("Data Type Out"=w571:T9, "Variant Out"=w570:variant)  [unwired: 11 in, 5 out]
                  n124 = case shown="\"I8\"..\"Extended Complex\"" w571 {
                    tunnel: w576 -> [w598 w605]
                    tunnel: w575 -> [w597 w604]
                    tunnel: [w598 w603] -> w574
                    tunnel: [w597 w602] -> w573
                    tunnel: w570 -> [_ w601]
                    tunnel: w565 -> [_ w599]
                    tunnel: w562 -> [_ w600]
                    frame Default {
                      # "Non-numeric data types will not\nhave any bearing on the execution time.\n\n--Ignore them"
                    }
                    frame "I8".."Extended Complex" {
                      # "Set the GFG with macro value"
                      # "Add to array if not present"
                      n125 = case shown="Default" w599 {
                        tunnel: w599 -> [w609 _]
                        tunnel: w600 -> [w608 _]
                        frame Default {
                          n126 = call "GFG_core.vi"("Variable Name in"=w609, "Variant in"=w608, "Action"=enum16{"Init", "Set", "Get", "Clear"}."Set") -> ()  [unwired: 10 in, 7 out]
                        }
                        frame "Laser.Power" {
                        }
                      }
                      n127 = Search 1D Array(1D array=w605, element=w599) -> (index of element=w607:i32)  [unwired: 1 in]
                      n128 = Greater Or Equal To 0?(x=w607) -> (x >= 0?=w606:bool)
                      n129 = case shown="False" w606 {
                        tunnel: w605 -> [w615 w617]
                        tunnel: w604 -> [w616 w618]
                        tunnel: [w614 w617] -> w603
                        tunnel: [w613 w618] -> w602
                        tunnel: w601 -> [w612 _]
                        tunnel: w599 -> [w611 _]
                        frame False {
                          n130 = Insert Into Array(array=w615, new element=w611) -> (w614:string[])  [unwired: 1 in]
                          n131 = Insert Into Array(array=w616, new element=w612) -> (w613:variant[])  [unwired: 1 in]
                        }
                        frame True {
                        }
                      }
                    }
                  }
                  n132 = case shown="False" w563 {
                    tunnel: w569 -> [w581 w596]
                    tunnel: w562 -> [w580 w595]
                    tunnel: w561 -> [w582 _]
                    tunnel: w560 -> [w579 _]
                    tunnel: [w578 w594] -> w559
                    frame False {
                      n133 = case shown="False" w582 {
                        tunnel: w581 -> [w585 w593]
                        tunnel: w580 -> [w584 w592]
                        tunnel: w579 -> [w586 _]
                        tunnel: [w583 w591] -> w578
                        frame False {
                          n134 = case shown="True" w586 {
                            tunnel: w585 -> [w587 w590]
                            tunnel: w584 -> [_ w589]
                            tunnel: [w587 w588] -> w583
                            frame False {
                            }
                            frame True {
                              n135 = Bundle By Name(cluster=w590, "Z"=w589) -> (w588:T7)
                            }
                          }
                        }
                        frame True {
                          n136 = Bundle By Name(cluster=w593, "Y"=w592) -> (w591:T7)
                        }
                      }
                    }
                    frame True {
                      n137 = Bundle By Name(cluster=w596, "X"=w595) -> (w594:T7)
                    }
                  }
                }
                n138 = Add(x=w552, y=w550) -> (x+y=w548:dbl)
                n139 = Insert Into Array(array=w551, new element=w550) -> (w549:dbl[])  [unwired: 1 in]
                n140 = Increment(x=w558) -> (x+1=w543:i32)
              }
              frame Default {
                w622 = inf
                # "Unknown command"
                n141 = Add(x=w622, y=w623) -> (x+y=w619:dbl)
                n142 = Insert Into Array(array=w621, new element=w622) -> (w620:dbl[])  [unwired: 1 in]
                n143 = Increment(x=w627) -> (x+1=w626:i32)
              }
              frame "Pause" {
                # "compensation factor for pause"
                n144 = Index Array(array=w647, index (row)=0, index (col)=1 ("disabled index (col)")) -> (element=w644:string)
                n145 = Increment(x=w650) -> (x+1=w649:i32)
                n146 = Fract/Exp String To Number(string=w644) -> (number=w641:dbl)  [unwired: 3 in, 1 out]
                n147 = Add(x=w641, y=0.1 ("number")) -> (x+y=w637:dbl)
                n148 = Add(x=w637, y=w639) -> (x+y=w638:dbl)
                n149 = Insert Into Array(array=w635, new element=w637) -> (w636:dbl[])  [unwired: 1 in]
              }
              frame "Record" {
                # "Is external trigger enabled?\nIf YES, we cannot estimate the run time\nHence use INFINITY"
                # "Add an extra 14%"
                # "Time for a Frame"
                n150 = call-poly "GFGpolyGet.vi"("Variable Name in"="external.start.trigger.enable") -> ("Boolean Value OUT"=w657:bool)  [unwired: 9 in, 1 out]
                n151 = case shown="False" w657 {
                  tunnel: [w676 inf] -> w656
                  tunnel: w653 -> [w674 _]
                  tunnel: w652 -> [w673 _]
                  frame False {
                    n152 = call "Is Command within a Preset.vi"("Index of command"=w673, "Macro Array IN"=w674) -> ("Index of Preset.Start"=w672:i32, "Part of a Macro?"=w675:bool)  [unwired: 7 in, 1 out]
                    n153 = case shown="True" w675 {
                      tunnel: [w677 w688] -> w676
                      tunnel: w674 -> [_ w690]
                      tunnel: w672 -> [_ w687]
                      frame False {
                        n154 = call-poly "GFGpolyGet.vi"("Variable Name in"="frames.p.sec") -> ("Numeric"=w682:dbl)  [unwired: 8 in, 2 out]
                        n155 = Reciprocal(x=w682) -> (1/x=w680:dbl)
                        n156 = call-poly "GFGpolyGet.vi"("Variable Name in"="no. of frames to acquire") -> ("Numeric"=w681:dbl)  [unwired: 8 in, 2 out]
                        n157 = Multiply(x=w680, y=w681) -> (x*y=w679:dbl)
                        n158 = Multiply(x=w679, y=1.14) -> (x*y=w677:dbl)
                      }
                      frame True {
                        n159 = Add(x=w687, y=3) -> (x+y=w685:i32)
                        n160 = Index Array(array=w690, index=w685) -> (element=w689:string)
                        n161 = call "Calculate execution time for scans.vi"("Command string IN"=w689) -> ("Execution time"=w688:dbl)  [unwired: 9 in, 1 out]
                      }
                    }
                  }
                  frame True {
                  }
                }
                n162 = Increment(x=w670) -> (x+1=w669:i32)
                n163 = Add(x=w654, y=w656) -> (x+y=w655:dbl)
                n164 = Add(x=w655, y=w665) -> (x+y=w664:dbl)
                n165 = Insert Into Array(array=w662, new element=w655) -> (w663:dbl[])  [unwired: 1 in]
              }
              frame "2D.Frame.Scan" {
                # "Is external trigger enabled?\nIf YES, we cannot estimate the run time\nHence use INFINITY"
                # "Add an extra 14%"
                # "Time for a Frame"
                n166 = call-poly "GFGpolyGet.vi"("Variable Name in"="external.start.trigger.enable") -> ("Boolean Value OUT"=w698:bool)  [unwired: 9 in, 1 out]
                n167 = case shown="False" w698 {
                  tunnel: [w715 inf] -> w697
                  tunnel: w696 -> [w714 _]
                  frame False {
                    n168 = call "Calculate execution time for scans.vi"("Command string IN"=w714) -> ("Execution time"=w713:dbl)  [unwired: 9 in, 1 out]
                    n169 = Multiply(x=w713, y=1.14) -> (x*y=w715:dbl)
                  }
                  frame True {
                  }
                }
                n170 = Increment(x=w711) -> (x+1=w710:i32)
                n171 = Add(x=w694, y=w692) -> (x+y=w693:dbl)
                n172 = Add(x=w697, y=w693) -> (x+y=w695:dbl)
                n173 = Add(x=w695, y=w706) -> (x+y=w705:dbl)
                n174 = Insert Into Array(array=w703, new element=w695) -> (w704:dbl[])  [unwired: 1 in]
              }
              frame "2D.Line.Scan" {
                # "Is external trigger enabled?\nIf YES, we cannot estimate the run time\nHence use INFINITY"
                # "Add an extra 14%"
                # "Time for a Frame"
                n175 = call-poly "GFGpolyGet.vi"("Variable Name in"="external.start.trigger.enable") -> ("Boolean Value OUT"=w724:bool)  [unwired: 9 in, 1 out]
                n176 = Increment(x=w737) -> (x+1=w736:i32)
                n177 = case shown="False" w724 {
                  tunnel: [w741 inf] -> w723
                  tunnel: w722 -> [w739 _]
                  frame False {
                    n178 = call "Calculate execution time for scans.vi"("Command string IN"=w739) -> ("Execution time"=w740:dbl)  [unwired: 9 in, 1 out]
                    n179 = Multiply(x=w740, y=1.14) -> (x*y=w741:dbl)
                  }
                  frame True {
                  }
                }
                n180 = Add(x=w720, y=w718) -> (x+y=w719:dbl)
                n181 = Add(x=w719, y=w723) -> (x+y=w721:dbl)
                n182 = Add(x=w721, y=w732) -> (x+y=w731:dbl)
                n183 = Insert Into Array(array=w729, new element=w721) -> (w730:dbl[])  [unwired: 1 in]
              }
              frame "Z.Stack" {
                # "Is external trigger enabled?\nIf YES, we cannot estimate the run time\nHence use INFINITY"
                # "Add an extra 14%"
                # "Time for a Frame"
                n184 = call-poly "GFGpolyGet.vi"("Variable Name in"="external.start.trigger.enable") -> ("Boolean Value OUT"=w750:bool)  [unwired: 9 in, 1 out]
                n185 = case shown="False" w750 {
                  tunnel: [w765 inf] -> w748
                  tunnel: w749 -> [w768 _]
                  frame False {
                    n186 = call "Calculate execution time for scans.vi"("Command string IN"=w768) -> ("Execution time"=w767:dbl)  [unwired: 9 in, 1 out]
                    n187 = Multiply(x=1.14 ("y"), y=w767) -> (x*y=w765:dbl)
                  }
                  frame True {
                  }
                }
                n188 = Increment(x=w763) -> (x+1=w762:i32)
                n189 = Add(x=w746, y=w744) -> (x+y=w745:dbl)
                n190 = Add(x=w748, y=w745) -> (x+y=w747:dbl)
                n191 = Add(x=w747, y=w758) -> (x+y=w757:dbl)
                n192 = Insert Into Array(array=w755, new element=w747) -> (w756:dbl[])  [unwired: 1 in]
              }
              frame "Fast.Z" {
                # "Is external trigger enabled?\nIf YES, we cannot estimate the run time\nHence use INFINITY"
                # "Add an extra 14%"
                # "Time for a Frame"
                n193 = call-poly "GFGpolyGet.vi"("Variable Name in"="external.start.trigger.enable") -> ("Boolean Value OUT"=w776:bool)  [unwired: 9 in, 1 out]
                n194 = case shown="False" w776 {
                  tunnel: [w793 inf] -> w775
                  tunnel: w774 -> [w792 _]
                  frame False {
                    n195 = call "Calculate execution time for scans.vi"("Command string IN"=w792) -> ("Execution time"=w791:dbl)  [unwired: 9 in, 1 out]
                    n196 = Multiply(x=w791, y=1.14) -> (x*y=w793:dbl)
                  }
                  frame True {
                  }
                }
                n197 = Increment(x=w789) -> (x+1=w788:i32)
                n198 = Add(x=w772, y=w770) -> (x+y=w771:dbl)
                n199 = Add(x=w771, y=w775) -> (x+y=w773:dbl)
                n200 = Add(x=w773, y=w784) -> (x+y=w783:dbl)
                n201 = Insert Into Array(array=w781, new element=w773) -> (w782:dbl[])  [unwired: 1 in]
              }
              frame "LOOP.Start" {
                w796 = 0.1 ("new element/subarray")
                # "approx Execution time\nfor a LOOP.Start"
                # "Increment index"
                # "Insert loop details into index 0"
                # "Get no. of iterations from the arguments of LOOP.Start"
                n202 = Index Array(array=w807, index (row)=0, index (col)=1 ("disabled index (col)")) -> (element=w814:string)
                n203 = Decimal String To Number(string=w814) -> (number=w805:i32)  [unwired: 2 in, 1 out]
                n204 = Bundle By Name(cluster=T5 {"Index of LOOP.Start"=0, "Iteration Count Down"=0, "No of iterations (N)"=0} ("LOOP Control Cluster"), "Index of LOOP.Start"=w810, "Iteration Count Down"=w805, "No of iterations (N)"=w805) -> (w804:T5)
                n205 = Insert Into Array(array=w803, new element=w796) -> (w802:dbl[])  [unwired: 1 in]
                n206 = Increment(x=w810) -> (x+1=w809:i32)
                n207 = Add(x=w798, y=w796) -> (x+y=w797:dbl)
                n208 = Insert Into Array(array=w813, index=0, new element=w804) -> (w812:T5[])
              }
              frame "LOOP.End" {
                w818 = 0.1 ("new element/subarray")
                # "approx Execution time\nfor a LOOP.Start"
                # "Determine next index"
                # "completed iterations?"
                n209 = Index Array(array=w835, index=0) -> (element=w832:T5)
                n210 = Unbundle By Name(w832) -> ("Index of LOOP.Start"=w828:i32, "Iteration Count Down"=w837:i32)
                n211 = Insert Into Array(array=w825, new element=w818) -> (w824:dbl[])  [unwired: 1 in]
                n212 = Add(x=w820, y=w818) -> (x+y=w819:dbl)
                n213 = Decrement(x=w837) -> (x-1=w831:i32)
                n214 = Less Or Equal To 0?(x=w831) -> (x <= 0?=w836:bool)
                n215 = Bundle(cluster=w832, "Index of LOOP.Start"=w828, "Iteration Count Down"=w831) -> (w826:T5)  [unwired: 1 in]
                n216 = case shown="False" w836 {
                  tunnel: w835 -> [w844 w850]
                  tunnel: [w841 w849] -> w834
                  tunnel: w826 -> [w842 _]
                  tunnel: w830 -> [_ w846]
                  tunnel: [w839 w845] -> w829
                  tunnel: w828 -> [w840 _]
                  frame False {
                    n217 = Increment(x=w840) -> (x+1=w839:i32)
                    n218 = Replace Array Subset(array=w844, new element=w842, index=0) -> (w841:T5[])
                  }
                  frame True {
                    n219 = Increment(x=w846) -> (x+1=w845:i32)
                    n220 = Delete From Array(array=w850, length=1, index=0) -> (array with subset deleted=w849:T5[])  [unwired: 1 out]
                  }
                }
              }
              frame "Slow.Z" {
                w854 = 0.1 ("new element/subarray")
                # "approx Execution overhead"
                # "Determine next index"
                # "completed iterations?"
                n221 = Insert Into Array(array=w861, new element=w854) -> (w860:dbl[])  [unwired: 1 in]
                n222 = Add(x=w856, y=w854) -> (x+y=w855:dbl)
                n223 = Increment(x=w853) -> (x+1=w852:i32)
              }
              frame "Tiling" {
                w867 = 0.1 ("new element/subarray")
                # "approx Execution overhead"
                # "Determine next index"
                # "completed iterations?"
                n224 = Insert Into Array(array=w874, new element=w867) -> (w873:dbl[])  [unwired: 1 in]
                n225 = Add(x=w869, y=w867) -> (x+y=w868:dbl)
                n226 = Increment(x=w866) -> (x+1=w865:i32)
              }
              frame "Preset.End" {
                w880 = 0.1 ("new element/subarray")
                # "approx Execution overhead"
                # "Determine next index"
                # "completed iterations?"
                n227 = Insert Into Array(array=w887, new element=w880) -> (w886:dbl[])  [unwired: 1 in]
                n228 = Add(x=w882, y=w880) -> (x+y=w881:dbl)
                n229 = Increment(x=w879) -> (x+1=w878:i32)
              }
            }
          }
          frame True {
            # "Set Estimated Run Time"
            # "Reset all GFG variables that were changed"
            # "Fininshed running through all commands. Reset index to 0"
            n230 = for {
              tunnel: w894 -> [w904] mode=indexing
              tunnel: w893 -> [w902] mode=indexing
              n231 = call "GFG_core.vi"("Variable Name in"=w904, "Variant in"=w902, "Action"=enum16{"Init", "Set", "Get", "Clear"}."Set") -> ()  [unwired: 10 in, 7 out]
            }
          }
        }
      }
      frame "Preview" {
        # "Is the index in range?"
        n232 = Array Size(array=w920) -> (size(s)=w922:i32)
        n233 = Greater Or Equal?(x=w907, y=w922) -> (x >= y?=w921:bool)
        n234 = case shown="False" w921 {
          selector: w921 -> [w937 w965]
          tunnel: w920 -> [w940 _]
          tunnel: w908 -> [w939 w964]
          tunnel: [w938 ExecutionStatus."Exec Complete" ("Execution Status")] -> w919
          tunnel: [w934 w967] -> w918
          tunnel: w907 -> [w931 w967]
          tunnel: [w937 w965] -> w917
          tunnel: [w927 _] -> w916
          tunnel: [w935 w964] -> w910
          tunnel: [w926 _] -> w906
          tunnel: w905 -> [w925 _]
          frame False {
            # "Increment index to execute next command"
            # "Set the Index (listened in Macro GUI)"
            n235 = Index Array(array=w940, index=w931) -> (element=w936:string)
            n236 = call "Decompose Command String.vi"("Error In"=w939, "Command IN"=w936) -> ("Error Out"=w930:errorcluster, "Action"=w927:string)  [unwired: 6 in, 2 out]
            n237 = call "Macro Action String to Action and Settings Enum.vi"("error in (no error)"=w930, "Action String IN"=w927) -> ("error out"=w929:errorcluster, "Action Enum OUT"=w928:T8)  [unwired: 6 in, 2 out]
            n238 = case shown="\"2D.Frame.Scan\", \"2D.Line.Scan\", \"Move.To.Position\", \"Z.Stack\", \"Fast.Z\"" w928 {
              tunnel: [ExecutionStatus."Skip" ("Execution Status") ExecutionStatus."Skip" ("Execution Status") ExecutionStatus."Skip" ("Execution Status") w950] -> w938
              tunnel: w929 -> [w942 w945 w948 w954]
              tunnel: w936 -> [_ _ _ w953]
              tunnel: [w942 w945 w948 w952] -> w935
              tunnel: [w941 TRUE FALSE w951] -> w926
              tunnel: w925 -> [w941 _ _ w951]
              frame Default {
              }
              frame "Slow.Z", "Tiling" {
              }
              frame "Preset.End" {
              }
              frame "2D.Frame.Scan", "2D.Line.Scan", "Move.To.Position", "Z.Stack", "Fast.Z" {
                # "Set the Execution status to 'Instruction Available' only for instructions that needs to be previewed"
                n239 = case shown="False" w951 {
                  tunnel: w954 -> [w958 w963]
                  tunnel: w953 -> [w957 _]
                  tunnel: [w956 w963] -> w952
                  tunnel: [ExecutionStatus."Instruction Available" ("Execution Status") ExecutionStatus."Skip" ("Execution Status")] -> w950
                  frame False {
                    n240 = To Variant(anything=w957) -> (Variant=w959:variant)
                    n241 = call "GFG_core.vi"("Variable Name in"="MacroInstr" ("Source VI"), "Variant in"=w959, "error in (no error)"=w958, "Action"=enum16{"Init", "Set", "Get", "Clear"}."Set") -> ("error out"=w956:errorcluster)  [unwired: 9 in, 6 out]
                  }
                  frame True {
                    # "Skip if elemnt inside a\nPreset group"
                  }
                }
              }
            }
            n242 = call "GFG_core.vi"("Variable Name in"="MacroExecIndex", "Variant in"=w931, "Action"=enum16{"Init", "Set", "Get", "Clear"}."Set") -> ()  [unwired: 10 in, 7 out]
            n243 = Increment(x=w931) -> (x+1=w934:i32)
          }
          frame True {
            # "Index is out of range! -- Completed all available commands"
          }
        }
      }
    }
  }
  "Error Out" <- w26
  "Execution Complete?" <- w22
  "Paused?" <- w21
  "Pause Duration" <- w25
  "Skip?" <- w20
  "Current Command" <- w23
  "Execution Status" <- w15
  "Remaining/Estimated Run Time" <- w17
  "Step time array" <- w18
  n244 = Decrement(x=w24) -> (x-1=→"Current Execution Index":i32)
  n245 = Bundle("number"=w17, w18) -> (→"Estimated Timing cluster":cluster{"number":dbl, dbl[]})  [unwired: 1 in]
  n246 = case shown="False" w22 {
    tunnel: [w969 ExecutionStatus."Exec Complete" ("Execution Status")] -> _
    tunnel: w21 -> [w970 _]
    tunnel: w20 -> [w968 _]
    frame False {
      n247 = case shown="False" w970 {
        tunnel: [w971 ExecutionStatus."Exec Paused" ("Execution Status")] -> w969
        tunnel: w968 -> [w972 _]
        frame False {
          n248 = case shown="False" w972 {
            tunnel: [ExecutionStatus."Instruction Available" ("Execution Status") ExecutionStatus."Skip" ("Execution Status")] -> w971
            frame False {
            }
            frame True {
            }
          }
        }
        frame True {
        }
      }
    }
    frame True {
    }
  }
